vi "InitChannelConf.vi"(8 "error in":errorcluster, 10 "Channel Num":u32, 11 "CAN-NI":refnum<class "CAN-NI.lvclass">) -> (0 "error out":errorcluster, 3 "CAN-NI":refnum<class "CAN-NI.lvclass">)   [LabVIEW 2019, in "CAN-NI.lvlib" / "CAN-NI.lvclass"]
uses:
  CAN-NI.lvclass
  TypeDef/ChannelProperty.ctl
  CAN-Interface/TypeDef/Def-Termination.ctl
  CAN-Interface/TypeDef/Def-Transmit Mode.ctl
  CAN-Interface/TypeDef/Def-Protocol.ctl
  CAN-NI.lvclass/CAN-NI.ctl
  CAN-Interface/Class-Interface.lvclass
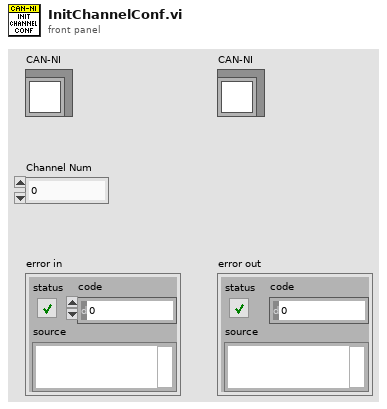
[diagram p1: front panel]
types:
  T1 = typedef "CAN-NI.lvlib/CAN-NI.lvclass/ChannelProperty.ctl" = cluster{"CAN-cluster":refnum<k21>, "CAN-Frames":refnum<k21>[], "Termination":T2, "Transmit Mode":T3, "Frame Out Session":refnum<k21>, "Frame In Session":refnum<k21>, "Protocol":T4}
  T2 = typedef "CAN-Interface.lvlib/Class-Interface.lvclass/Def-Termination.ctl" = enum8{"on", "off"}
  T3 = typedef "CAN-Interface.lvlib/Class-Interface.lvclass/Def-Transmit Mode.ctl" = enum16{"Queued", "Stream"}
  T4 = typedef "CAN-Interface.lvlib/Class-Interface.lvclass/Def-Protocol.ctl" = enum16{"CAN", "CAN FD"}
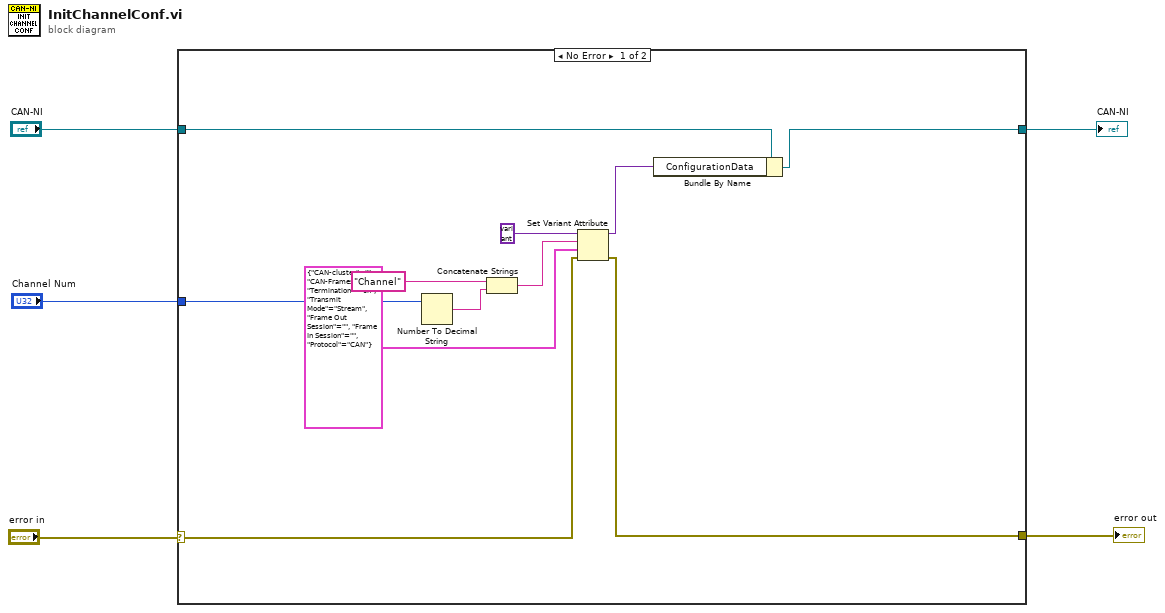
[diagram p0: block diagram]
diagram:
  n1 = case shown="No Error" "error in" {
    selector: "error in" -> [w7 w17]
    tunnel: "CAN-NI" -> [w10 w18]
    tunnel: "Channel Num" -> [w11 _]
    tunnel: [w9 w18] -> w2
    tunnel: [w6 w17] -> w1
    frame No Error {
      n2 = Number To Decimal String(number=w11) -> (decimal integer string=w15:string)  [unwired: 1 in]
      n3 = Concatenate Strings("Channel" ("string"), w15) -> (w16:string)
      n4 = Set Variant Attribute(Variant=variant, name=w16, value=T1 {"CAN-cluster"="", "CAN-Frames"=[], "Termination"=enum."on", "Transmit Mode"=enum."Stream", "Frame Out Session"="", "Frame In Session"="", "Protocol"=enum."CAN"} ("ChannelProperty"), error in=w7) -> (Variant out=w8:variant, error out=w6:errorcluster)  [unwired: 1 out]
      n5 = Bundle By Name(cluster=w10, "ConfigurationData"=w8) -> (w9:refnum<class "CAN-NI.lvclass">)
    }
    frame Error {
    }
  }
  "CAN-NI" <- w2
  "error out" <- w1
